vi "ResetCount.vi"(8 "error in (no error)":errorcluster, 11 "TopLevel in":refnum<class "TopLevel.lvclass">) -> (0 "error out":errorcluster, 3 "TopLevel out":refnum<class "TopLevel.lvclass">)   [LabVIEW 2019, in "TopLevel.lvlib" / "TopLevel.lvclass"]
uses:
  TopLevel.lvclass
  TopLevel.lvclass/TopLevel.ctl
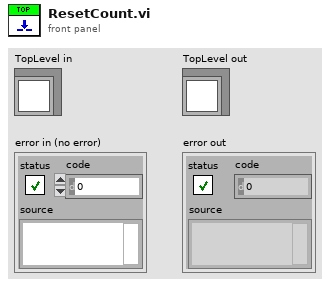
[diagram p1: front panel]
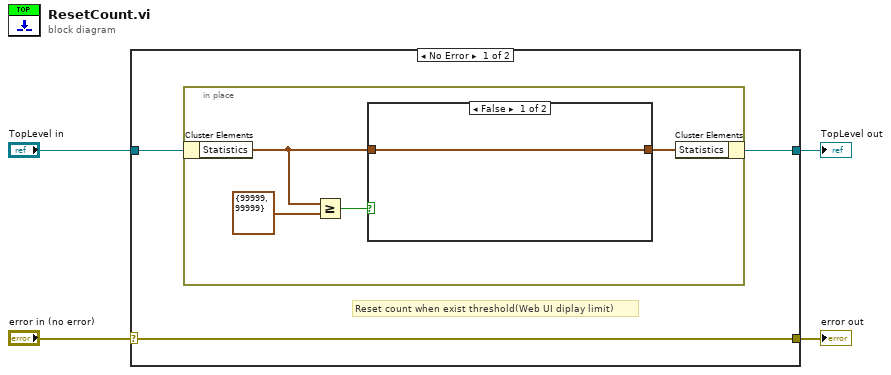
[diagram p0: block diagram]
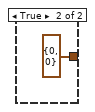
[diagram p2: hidden frame]
diagram:
  n1 = case shown="No Error" "error in (no error)" {
    selector: "error in (no error)" -> [w5 w15]
    tunnel: [w5 w15] -> w3
    tunnel: [w6 w14] -> w1
    tunnel: "TopLevel in" -> [w7 w14]
    frame No Error {
      # "Reset count when exist threshold(Web UI diplay limit)"
      n2 = in-place {
        n3 = in-place-cluster #1(w7) -> ("Statistics"=w9:cluster{"OK":i32, "NG":i32})
        n4 = Greater Or Equal?(x=w9, y=cluster{"OK":i32, "NG":i32} {"OK"=99999, "NG"=99999}) -> (x >= y?=w10:bool)
        n5 = case shown="False" w10 {
          tunnel: w9 -> [w12 _]
          tunnel: [w12 cluster{"OK":i32, "NG":i32} {"OK"=0, "NG"=0} ("Statistics")] -> w8
          frame False {
          }
          frame True {
          }
        }
        n6 = in-place-cluster #1("Statistics"=w8) -> (w6:refnum<class "TopLevel.lvclass">)
      }
    }
    frame Error {
    }
  }
  "error out" <- w3
  "TopLevel out" <- w1
